vi "piddesposito.vi"() -> ()   [LabVIEW 2015]
panel:
  in  "Cluster":cluster{}
  in  "Abierto":bool
  in  "Disminuir":bool
  out "Tank":dbl(slide) scale=0.0..200.0
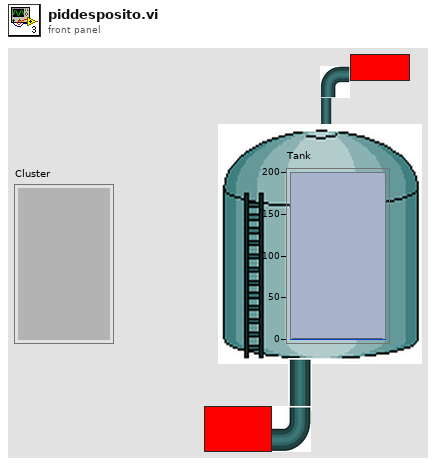
[diagram p1: front panel]
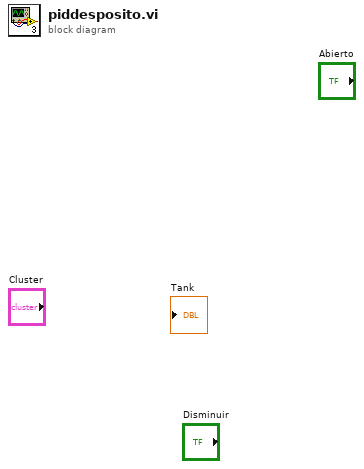
[diagram p0: block diagram]
diagram:
